vi "Monitor.vi"(0 "Temp.Max":dbl, 1 "Temp.Min":dbl, 2 "User name input":string, 3 "error in (no error)":errorcluster, 4 "Time/Date":timestamp) -> (5 "History Data":T1, 6 "error out":errorcluster)   [LabVIEW 2021]
doc: "Mide la temperatura del sensor de temperatura de una DAQ mientras regula que esa temperatura se mantenga dentro de los límites establecidos por Temp.Max y Temp.Min"
uses:
  Controles/Estados Monitor.ctl
panel:
  out "Heater Level (V)":dbl format="%_3g"
  in  "QUIT":bool
  in  "Stop":bool
  in  "Start":bool
  out "VENTILATOR":bool
  out "HEATER":string
  out "Temp (ºC)":dbl(slide) scale=0.0..100.0
  out "Temperature Data":T2(graph)={"Temp.Max"=27.3, "RTD Temp"=21.528194944839925, "Temp.Min"=27.1}
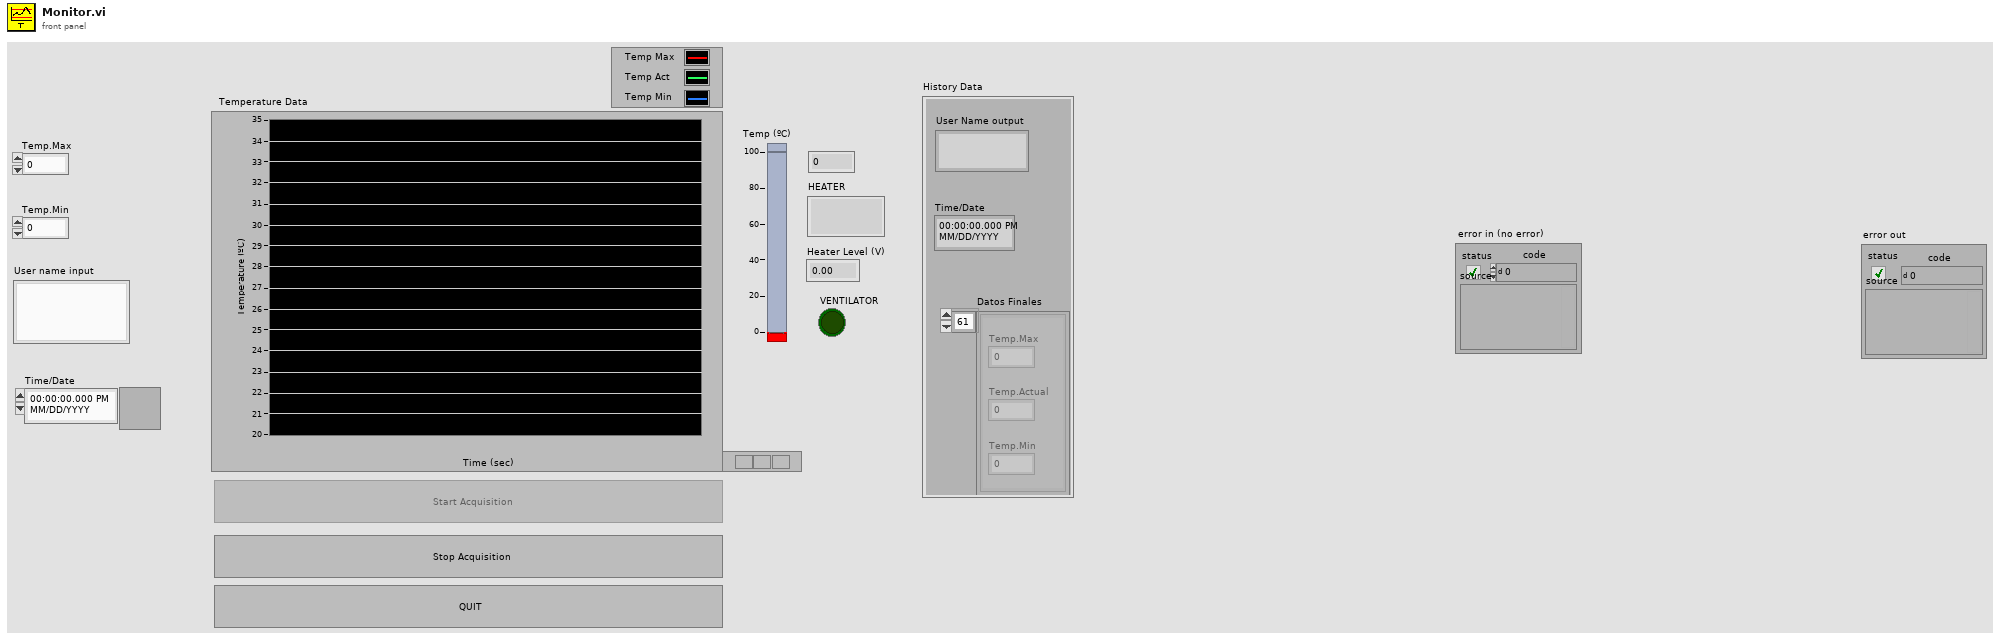
[diagram p1: front panel]
types:
  T1 = cluster{"User Name output":string, "Time/Date":timestamp, "Datos Finales":cluster{"Temp.Max":dbl, "Temp.Actual":dbl, "Temp.Min":dbl}[]}
  T2 = cluster{"Temp.Max":dbl, "RTD Temp":dbl, "Temp.Min":dbl}
  T3 = enum8{"Enabled", "Disabled", "Disabled and Grayed Out"}
  T4 = cluster{"Temp.Max":dbl, "Temp.Actual":dbl, "Temp.Min":dbl}[]
  T5 = cluster{"Temp.Max":dbl, "Temp.Min":dbl, "Temp.Actual":dbl}[]
  T6 = typedef "Estados Monitor.ctl" = enum16{"Initialize", "Measure", "Cooling", "Maximum", "Medium", "View Acquired Data", "Quit"}
  T7 = cluster{"Temp.Max OUT":dbl, "RTD Temp":dbl, "Temp.Min OUT":dbl}
  T8 = cluster{"User name input":string, "Time/Date":timestamp, "Datos Finales":cluster{"Temp.Max":dbl, "Temp.Min":dbl, "Temp.Actual":dbl}[]}
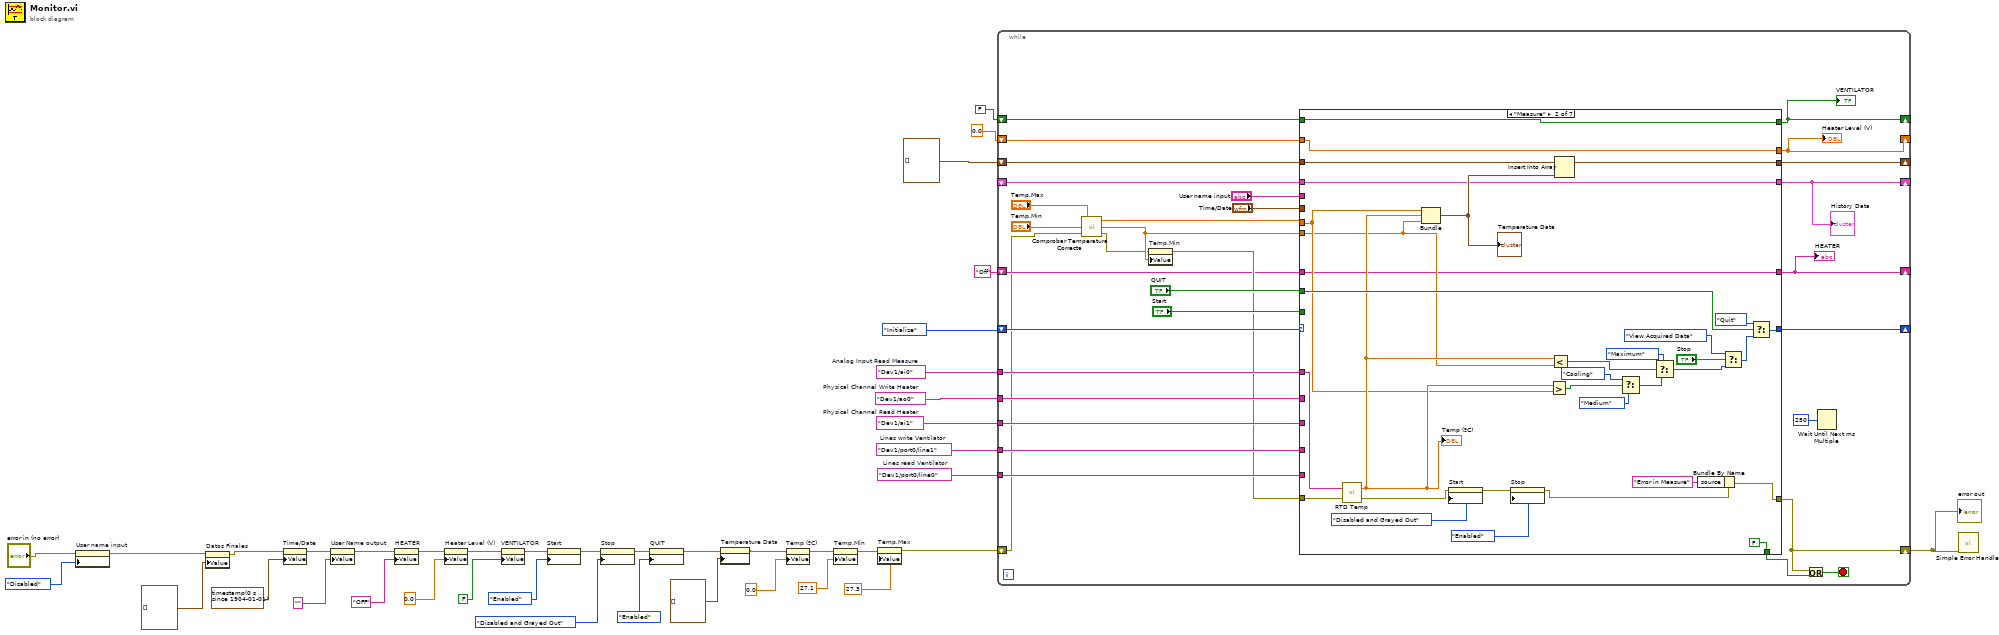
[diagram p0: block diagram]
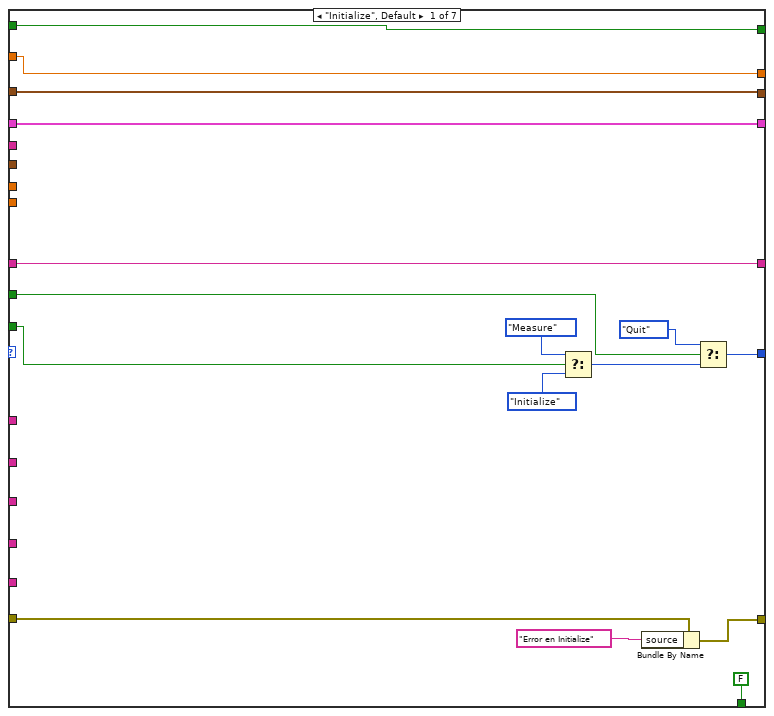
[diagram p2: hidden frame]
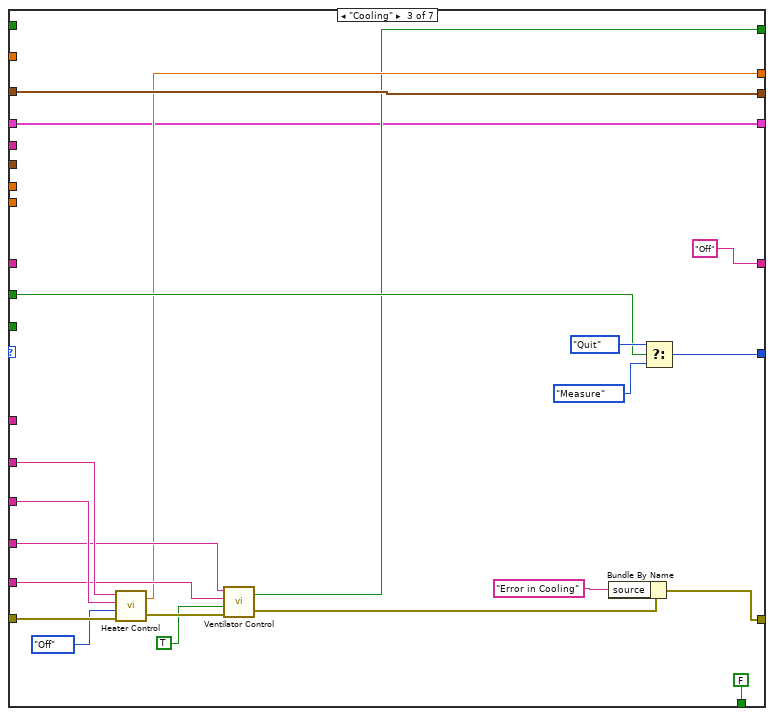
[diagram p3: hidden frame]
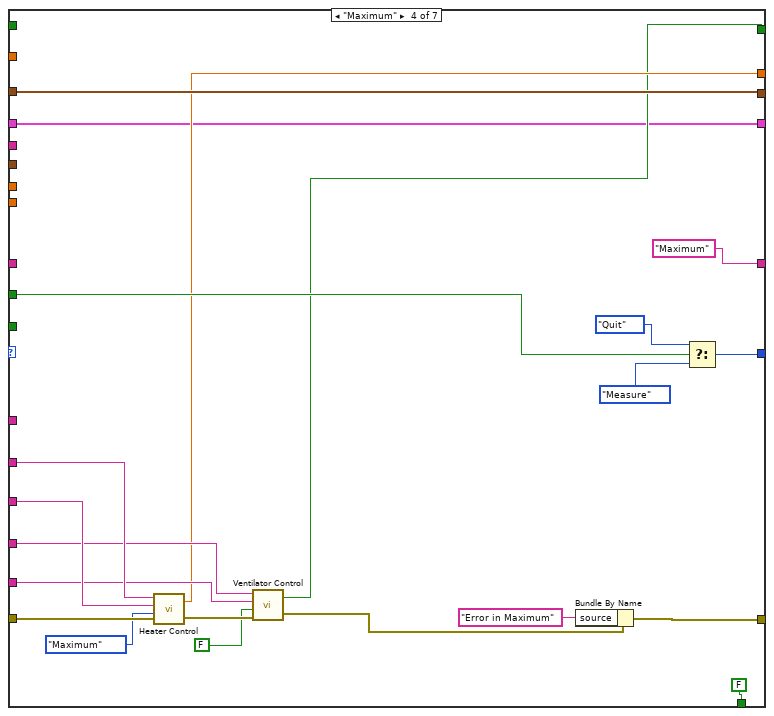
[diagram p4: hidden frame]
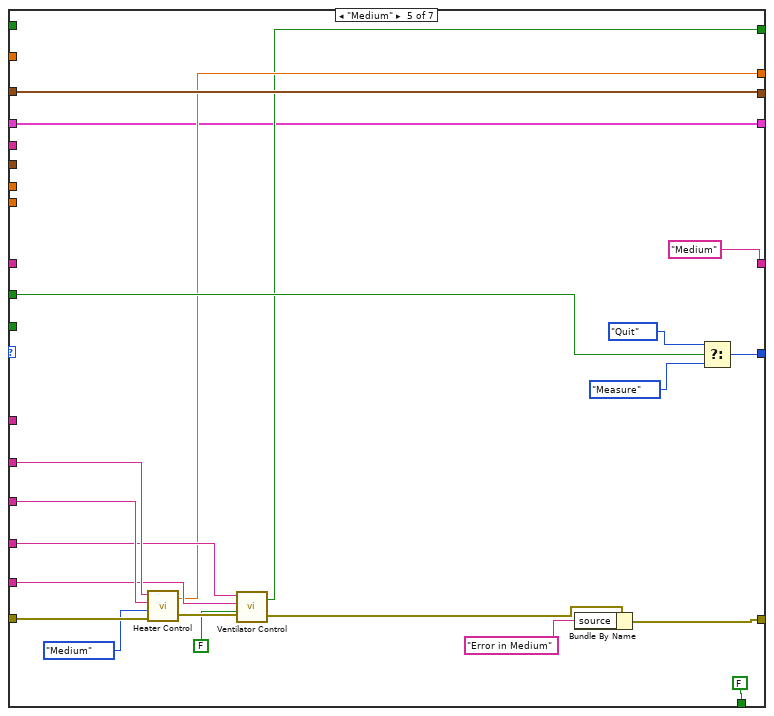
[diagram p5: hidden frame]
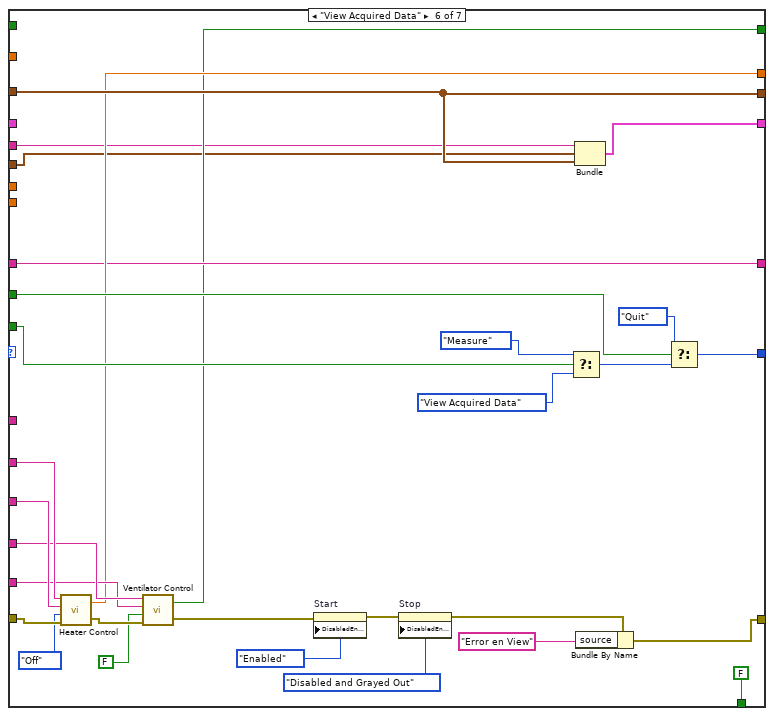
[diagram p6: hidden frame]
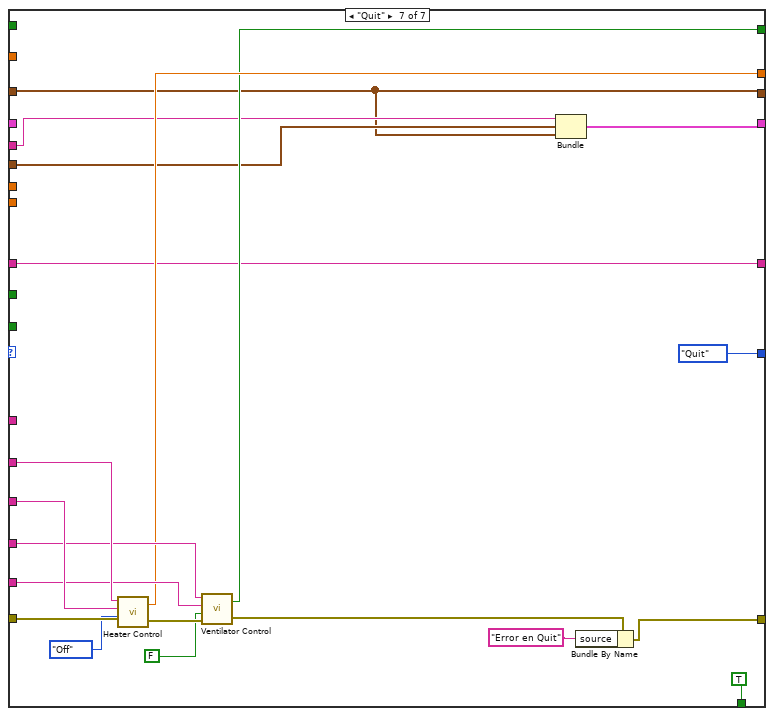
[diagram p7: hidden frame]
diagram:
  w9 = tag "Dev1/port0/line1"  # Lines write Ventilator
  w8 = tag "Dev1/port0/line0"  # Lines read Ventilator
  w7 = tag "Dev1/ai1"  # Physical Channel Read Heater
  w6 = tag "Dev1/ao0"  # Physical Channel Write Heater
  w5 = tag "Dev1/ai0"  # Analog Input Read Measure
  n1 = property on="User name input" class="Str"(error in="error in (no error)", "DisabledEnum"=T3."Disabled" ("Disabled")) -> (error out=w1:errorcluster)  [unwired: 1 in, 1 out]
  n2 = property on="Datos Finales" class="Arr (strict)"(error in=w1, "Value"=T4 [] ("Datos Finales")) -> (error out=w14:errorcluster)  [unwired: 1 in, 1 out]
  n3 = property on="Time/Date" class="AbsTime (strict)"(error in=w14, "Value"=timestamp(0 s since 1904-01-01) ("Time/Date")) -> (error out=w38:errorcluster)  [unwired: 1 in, 1 out]
  n4 = property on="User Name output" class="Str"(error in=w38, "Value"="" ("User Name")) -> (error out=w36:errorcluster)  [unwired: 1 in, 1 out]
  n5 = property on="HEATER" class="Str"(error in=w36, "Value"="OFF" ("HEATER")) -> (error out=w34:errorcluster)  [unwired: 1 in, 1 out]
  n6 = property on="Heater Level (V)" class="DigNum (strict)"(error in=w34, "Value"=0.0 ("Heater Level (V)")) -> (error out=w32:errorcluster)  [unwired: 1 in, 1 out]
  n7 = property on="VENTILATOR" class="Bool (strict)"(error in=w32, "Value"=FALSE ("VENTILATOR")) -> (error out=w28:errorcluster)  [unwired: 1 in, 1 out]
  n8 = property on="Start" class="Bool"(error in=w28, "DisabledEnum"=T3."Enabled" ("Disabled")) -> (error out=w27:errorcluster)  [unwired: 1 in, 1 out]
  n9 = property on="Stop" class="Bool"(error in=w27, "DisabledEnum"=T3."Disabled and Grayed Out" ("Disabled")) -> (error out=w26:errorcluster)  [unwired: 1 in, 1 out]
  n10 = property on="QUIT" class="Bool"(error in=w26, "DisabledEnum"=T3."Enabled" ("Disabled")) -> (error out=w13:errorcluster)  [unwired: 1 in, 1 out]
  n11 = property on="Temperature Data" class="WFChart (strict)"(error in=w13, "History Data"=T4 [] ("Datos Finales")) -> (error out=w12:errorcluster)  [unwired: 1 in, 1 out]
  n12 = property on="Temp (ºC)" class="Slide (strict)"(error in=w12, "Value"=0.0 ("Temp (ºC)")) -> (error out=w23:errorcluster)  [unwired: 1 in, 1 out]
  n13 = property on="Temp.Min" class="DigNum (strict)"(error in=w23, "Value"=27.1 ("Temp.Min")) -> (error out=w22:errorcluster)  [unwired: 1 in, 1 out]
  n14 = property on="Temp.Max" class="DigNum (strict)"(error in=w22, "Value"=27.3 ("Temp.Max")) -> (error out=w21:errorcluster)  [unwired: 1 in, 1 out]
  n15 = while {
    shift-right: [w68] -> _
    shift-left: Estados_Monitor."Initialize" ("Estados Monitor") -> [w72]
    shift-right: [w70] -> w10
    shift-left: w21 -> [w42]
    shift-right: [w65] -> _
    shift-left: FALSE ("Ventilator State") -> [w62]
    shift-right: [w64] -> _
    shift-left: 0.0 ("Heater Level (V)") -> [w63]
    shift-right: [w60] -> _
    shift-left: T5 [] ("Datos Finales") -> [w61]
    tunnel: w9 -> [w58]
    tunnel: w8 -> [w57]
    tunnel: w7 -> [w56]
    tunnel: w6 -> [w55]
    tunnel: w5 -> [w54]
    shift-right: [w52] -> _
    shift-left: "Off" ("HEATER") -> [w51]
    shift-right: [w47] -> _
    shift-left: _ -> [w48]
    stop <- w71 stop-if-true
    n16 = call "Comprobar Temperatura Correcta.vi"("error in (no error)"=w42, "Temp.Min IN"="Temp.Min", "Temp.Max  IN"="Temp.Max") -> ("error out"=w41:errorcluster, "Temp.Min OUT"=w43:dbl, "Temp.Max OUT"=w44:dbl)
    n17 = property on="Temp.Min" class="DigNum (strict)"(error in=w41, "Value"=w43) -> (error out=w53:errorcluster)  [unwired: 1 in, 1 out]
    n18 = case shown="\"Measure\"" w72 {
      tunnel: w53 -> [w87 w120 w142 w163 w184 w199 w233]
      tunnel: [FALSE ("x") FALSE ("x") FALSE ("x") FALSE ("x") FALSE ("x") FALSE ("x") TRUE] -> w69
      tunnel: [w85 w106 w138 w158 w180 w213 w229] -> w70
      tunnel: [w79 w107 w132 w153 w174 w201 Estados_Monitor."Quit" ("Estados Monitor")] -> w68
      tunnel: "QUIT" -> [w82 w110 w126 w156 w177 w202 _]
      tunnel: [w76 w91 w124 w146 w167 w188 w220] -> w65
      tunnel: [w78 w92 w125 w147 w168 w191 w221] -> w64
      tunnel: w63 -> [w78 w92 _ _ _ _ _]
      tunnel: w62 -> [w76 w91 _ _ _ _ _]
      tunnel: w61 -> [w77 w98 w131 w152 w173 w200 w216]
      tunnel: [w77 w96 w131 w152 w173 w200 w216] -> w60
      tunnel: "Start" -> [w75 _ _ _ _ w207 _]
      tunnel: w54 -> [_ w95 _ _ _ _ _]
      tunnel: w55 -> [_ _ w130 w150 w171 w197 w225]
      tunnel: w56 -> [_ _ w129 w151 w172 w196 w224]
      tunnel: w57 -> [_ _ w128 w148 w169 w193 w222]
      tunnel: w58 -> [_ _ w127 w149 w170 w194 w223]
      tunnel: w44 -> [_ w94 _ _ _ _ _]
      tunnel: w43 -> [_ w93 _ _ _ _ _]
      tunnel: [w74 w90 "Off" ("HEATER") "Maximum" ("HEATER") "Medium" ("HEATER") w190 w219] -> w52
      tunnel: w51 -> [w74 w90 _ _ _ w190 w219]
      tunnel: "User name input" -> [_ _ _ _ _ w187 w218]
      tunnel: "Time/Date" -> [_ _ _ _ _ w186 w217]
      tunnel: [w73 w89 w122 w143 w164 w185 w215] -> w47
      tunnel: w48 -> [w73 w89 w122 w143 w164 _ _]
      frame "Initialize", Default {
        n19 = Select(t=Estados_Monitor."Measure" ("Estados Monitor"), s=w75, f=Estados_Monitor."Initialize" ("Estados Monitor")) -> (s? t:f=w80:T6)
        n20 = Bundle By Name(cluster=w87, "source"="Error en Initialize") -> (w85:errorcluster)
        n21 = Select(t=Estados_Monitor."Quit" ("Estados Monitor"), s=w82, f=w80) -> (s? t:f=w79:T6)
      }
      frame "Measure" {
        n22 = call "RTD Temp.vi"("error in (no error)"=w120, "DAQmx Physical Channel"=w95) -> ("error out"=w101:errorcluster, "RTD Temp"=w104:dbl)
        "Temp (ºC)" <- w104
        n23 = Bundle("Temp.Max OUT"=w94, "RTD Temp"=w104, "Temp.Min OUT"=w93) -> (w97:T7)  [unwired: 1 in]
        "Temperature Data" <- w97
        n24 = property on="Start" class="Bool"(error in=w101, "DisabledEnum"=T3."Disabled and Grayed Out" ("Disabled")) -> (error out=w100:errorcluster)  [unwired: 1 in, 1 out]
        n25 = property on="Stop" class="Bool"(error in=w100, "DisabledEnum"=T3."Enabled" ("Disabled")) -> (error out=w99:errorcluster)  [unwired: 1 in, 1 out]
        n26 = Greater?(x=w104, y=w94) -> (0:w119:bool)
        n27 = Less?(x=w104, y=w93) -> (x < y?=w116:bool)
        n28 = Insert Into Array(array=w98, new element=w97) -> (w96:T5)  [unwired: 1 in]
        n29 = Select(t=Estados_Monitor."Cooling" ("Estados Monitor"), s=w119, f=Estados_Monitor."Medium" ("Estados Monitor")) -> (s? t:f=w114:T6)
        n30 = Select(t=Estados_Monitor."Maximum" ("Estados Monitor"), s=w116, f=w114) -> (s? t:f=w111:T6)
        n31 = Bundle By Name(cluster=w99, "source"="Error in Measure") -> (w106:errorcluster)
        n32 = Select(t=Estados_Monitor."View Acquired Data" ("Estados Monitor"), s="Stop", f=w111) -> (s? t:f=w108:T6)
        n33 = Select(t=Estados_Monitor."Quit" ("Estados Monitor"), s=w110, f=w108) -> (s? t:f=w107:T6)
      }
      frame "Cooling" {
        n34 = call "Heater Control.vi"("error in (no error)"=w142, "Heater Level"=enum16{"Off", "Medium", "Maximum"}."Off", "Physical Channel Read"=w129, "Physical Channel Write"=w130) -> ("error out"=w141:errorcluster, "Heater Level (V)"=w125:dbl)
        n35 = call "Ventilator Control.vi"("error in (no error)"=w141, "Ventilator (off)"=TRUE, "Lines read"=w128, "Lines write"=w127) -> ("error out"=w139:errorcluster, "Ventilator State"=w124:bool)
        n36 = Bundle By Name(cluster=w139, "source"="Error in Cooling") -> (w138:errorcluster)
        n37 = Select(t=Estados_Monitor."Quit" ("Estados Monitor"), s=w126, f=Estados_Monitor."Measure" ("Estados Monitor")) -> (s? t:f=w132:T6)
      }
      frame "Maximum" {
        n38 = call "Heater Control.vi"("error in (no error)"=w163, "Heater Level"=enum16{"Off", "Medium", "Maximum"}."Maximum", "Physical Channel Read"=w151, "Physical Channel Write"=w150) -> ("error out"=w161:errorcluster, "Heater Level (V)"=w147:dbl)
        n39 = call "Ventilator Control.vi"("error in (no error)"=w161, "Ventilator (off)"=FALSE, "Lines read"=w148, "Lines write"=w149) -> ("error out"=w145:errorcluster, "Ventilator State"=w146:bool)
        n40 = Bundle By Name(cluster=w145, "source"="Error in Maximum") -> (w158:errorcluster)
        n41 = Select(t=Estados_Monitor."Quit" ("Estados Monitor"), s=w156, f=Estados_Monitor."Measure" ("Estados Monitor")) -> (s? t:f=w153:T6)
      }
      frame "Medium" {
        n42 = call "Heater Control.vi"("error in (no error)"=w184, "Heater Level"=enum16{"Off", "Medium", "Maximum"}."Medium", "Physical Channel Read"=w172, "Physical Channel Write"=w171) -> ("error out"=w183:errorcluster, "Heater Level (V)"=w168:dbl)
        n43 = call "Ventilator Control.vi"("error in (no error)"=w183, "Ventilator (off)"=FALSE, "Lines read"=w169, "Lines write"=w170) -> ("error out"=w166:errorcluster, "Ventilator State"=w167:bool)
        n44 = Bundle By Name(cluster=w166, "source"="Error in Medium") -> (w180:errorcluster)
        n45 = Select(t=Estados_Monitor."Quit" ("Estados Monitor"), s=w177, f=Estados_Monitor."Measure" ("Estados Monitor")) -> (s? t:f=w174:T6)
      }
      frame "View Acquired Data" {
        n46 = call "Heater Control.vi"("error in (no error)"=w199, "Heater Level"=enum16{"Off", "Medium", "Maximum"}."Off", "Physical Channel Read"=w196, "Physical Channel Write"=w197) -> ("error out"=w198:errorcluster, "Heater Level (V)"=w191:dbl)
        n47 = call "Ventilator Control.vi"("error in (no error)"=w198, "Ventilator (off)"=FALSE, "Lines read"=w193, "Lines write"=w194) -> ("error out"=w189:errorcluster, "Ventilator State"=w188:bool)
        n48 = property on="Start" class="Bool"(error in=w189, "DisabledEnum"=T3."Enabled" ("Disabled")) -> (error out=w209:errorcluster)  [unwired: 1 in, 1 out]
        n49 = property on="Stop" class="Bool"(error in=w209, "DisabledEnum"=T3."Disabled and Grayed Out" ("Disabled")) -> (error out=w208:errorcluster)  [unwired: 1 in, 1 out]
        n50 = Select(t=Estados_Monitor."Measure" ("Estados Monitor"), s=w207, f=Estados_Monitor."View Acquired Data" ("Estados Monitor")) -> (s? t:f=w203:T6)
        n51 = Bundle("User name input"=w187, "Time/Date"=w186, "Datos Finales"=w200) -> (w185:T8)  [unwired: 1 in]
        n52 = Bundle By Name(cluster=w208, "source"="Error en View") -> (w213:errorcluster)
        n53 = Select(t=Estados_Monitor."Quit" ("Estados Monitor"), s=w202, f=w203) -> (s? t:f=w201:T6)
      }
      frame "Quit" {
        n54 = call "Heater Control.vi"("error in (no error)"=w233, "Heater Level"=enum16{"Off", "Medium", "Maximum"}."Off", "Physical Channel Read"=w224, "Physical Channel Write"=w225) -> ("error out"=w231:errorcluster, "Heater Level (V)"=w221:dbl)
        n55 = call "Ventilator Control.vi"("error in (no error)"=w231, "Ventilator (off)"=FALSE, "Lines read"=w222, "Lines write"=w223) -> ("error out"=w230:errorcluster, "Ventilator State"=w220:bool)
        n56 = Bundle("User name input"=w218, "Time/Date"=w217, "Datos Finales"=w216) -> (w215:T8)  [unwired: 1 in]
        n57 = Bundle By Name(cluster=w230, "source"="Error en Quit") -> (w229:errorcluster)
      }
    }
    "VENTILATOR" <- w65
    "Heater Level (V)" <- w64
    "HEATER" <- w52
    "History Data" <- w47
    n58 = Or(x=w70, y=w69) -> (x .or. y?=w71:bool)
    n59 = Wait Until Next ms Multiple(millisecond multiple=u32 250 ("millisecond timer value")) -> ()  [unwired: 1 out]
  }
  "error out" <- w10
  n60 = call <vilib>:"Simple Error Handler.vi"("error in (no error)"=w10) -> ()  [unwired: 4 in, 5 out]
